vi "TRITON_PARSE_PRESSURE.vi"(2 "Pressures String":string) -> ()   [LabVIEW 2009]
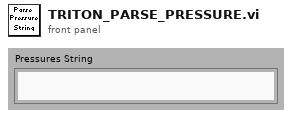
[diagram p1: front panel]
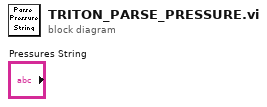
[diagram p0: block diagram]
diagram:
